vi "character_condition.vi"() -> ()   [LabVIEW 2021]
panel:
  out "Array":bool[](array[boolean])
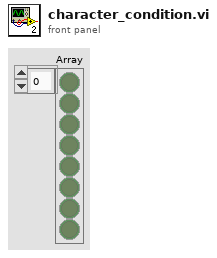
[diagram p1: front panel]
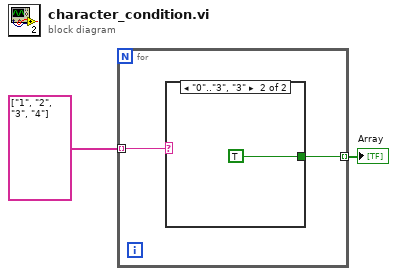
[diagram p0: block diagram]
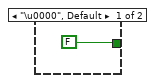
[diagram p2: hidden frame]
diagram:
  n1 = for {
    tunnel: string[] ["1", "2", "3", "4"] -> [w4] mode=indexing
    tunnel: [w3] -> w1 mode=indexing
    n2 = case shown="\"0\"..\"3\", \"3\"" w4 {
      tunnel: [FALSE TRUE] -> w3
      frame "\u0000", Default {
      }
      frame "0".."3", "3" {
      }
    }
  }
  "Array" <- w1
